vi "Write GUID.vi"(6 "GUID":string, 11 "ITest Executive Builder Dialog in":refnum<class "ITest Executive Builder Dialog.lvclass">) -> (3 "ITest Executive Builder Dialog out":refnum<class "ITest Executive Builder Dialog.lvclass">)   [LabVIEW 2017, in "ITest Executive Builder Dialog.lvclass"]
uses:
  <vilib>/gpm_packages/@cs/Test-executive-builder/Source/Test Executive Builder Dialogs/ITest Executive Builder Dialog/ITest Executive Builder Dialog.lvclass
  <vilib>/gpm_packages/@cs/Test-executive-builder/Source/Test Executive Builder Dialogs/ITest Executive Builder Dialog/ITest Executive Builder Dialog.lvclass/ITest Executive Builder Dialog.ctl
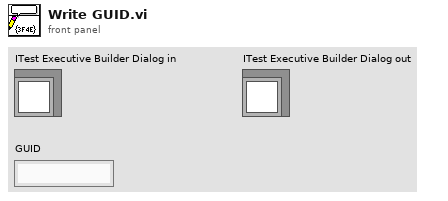
[diagram p1: front panel]
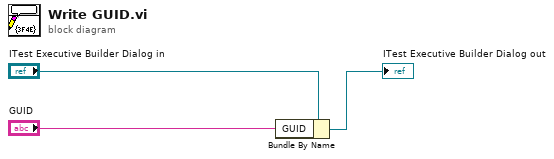
[diagram p0: block diagram]
diagram:
  n1 = Bundle By Name(cluster="ITest Executive Builder Dialog in", "GUID"="GUID") -> (→"ITest Executive Builder Dialog out":refnum<class "ITest Executive Builder Dialog.lvclass">)
